vi "Get MDIF Blocks (Block Name).vi"(8 "error in (no error)":errorcluster, 10 "Block Name":string, 11 "MDIF reference in":refnum<k24>) -> (0 "error out":errorcluster, 2 "MDIF Blocks":T1[](array[typedef]), 3 "MDIF reference out":refnum<k24>)   [LabVIEW 2023, in "NI_HFNetworkAnalysis.lvlib"]
doc: "Retrieve the MDIF block in memory with the specified <b>Block Name</b> for the referenced MDIF file."
uses:
  NI_HFNetworkAnalysis.lvlib
  C:/srd-semi-rfcal-software/AuxTools/STSRFFixtureCharactUtility/Source/Code Modules/Fixture/Dependencies/HFNetworkAnalysis/Support Files/NACE.Utils.Data.dll
  Support Files/NACE.Utils.Data.dll
  Controls/MDIF Block.ctl
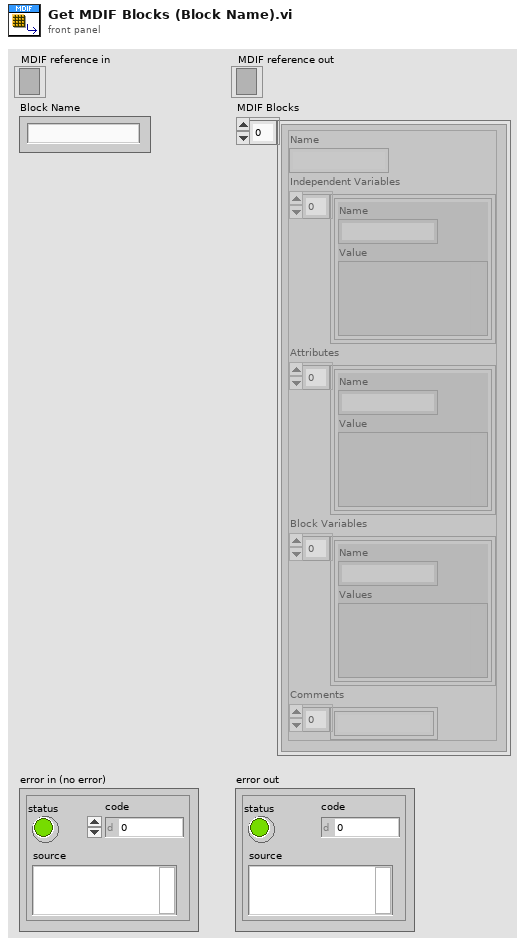
[diagram p1: front panel]
types:
  T1 = typedef "NI_HFNetworkAnalysis.lvlib/MDIF Block.ctl" = cluster{"Name":string, "Independent Variables":cluster{"Name":string, "Value":variant}[], "Attributes":cluster{"Name":string, "Value":variant}[], "Block Variables":cluster{"Name":string, "Values":variant}[], "Comments":string[]}
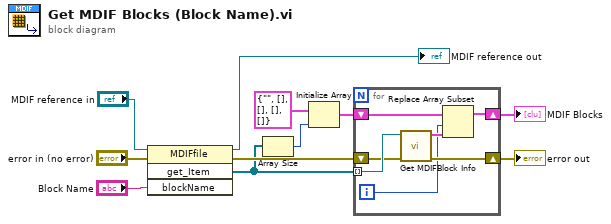
[diagram p0: block diagram]
diagram:
  n1 = invoke class="MDIFfile" method="get_Item"(reference="MDIF reference in", error in="error in (no error)", "blockName"="Block Name") -> (reference out=→"MDIF reference out":refnum<k24>, error out=w11:errorcluster, "get_Item"=w3:refnum<k24>[])  [unwired: 1 in, 1 out]
  n2 = Array Size(array=w3) -> (size(s)=w4:i32)
  n3 = Initialize Array(T1 {"Name"="", "Independent Variables"=[], "Attributes"=[], "Block Variables"=[], "Comments"=[]} ("MDIF Block"), w4) -> (w2:T1[])
  n4 = for {
    shift-right: [w18] -> w8
    shift-left: w11 -> [w16]
    tunnel: w3 -> [w17] mode=indexing
    shift-right: [w12] -> w1
    shift-left: w2 -> [w15]
    i -> [w13]
    n5 = call "Get MDIFBlock Info.vi"("error in (no error)"=w16, "MDIF Block Refnum in"=w17) -> ("error out"=w18:errorcluster, "MDIF Block"=w14:T1)  [unwired: 8 in]
    n6 = Replace Array Subset(array=w15, new element=w14, index=w13) -> (w12:T1[])
  }
  "MDIF Blocks" <- w1
  "error out" <- w8
